vi "TracePointSetSystemTime.vi"() -> (1 "tracepoint name":string)   [LabVIEW 2017, in "DeviceHealth.lvlib"]
uses:
  <vilib>/addons/InsightCM/Devices/Shared/Common/DeviceHealth/DeviceHealth.lvlib
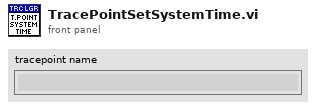
[diagram p1: front panel]
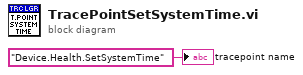
[diagram p0: block diagram]
diagram:
  "tracepoint name" <- "Device.Health.SetSystemTime" ("ProcessName")
